vi "GUITest.vi"() -> ()   [LabVIEW 2021]
uses:
  <vilib>/Analysis/1siggen.llb/Ramp Pattern by Samples.vi
  <vilib>/Analysis/NI_AALBase.lvlib
panel:
  out "XY Graph":T1(graph)
  out "element":dbl
  out "Ramp Pattern":dbl[](array[numeric])
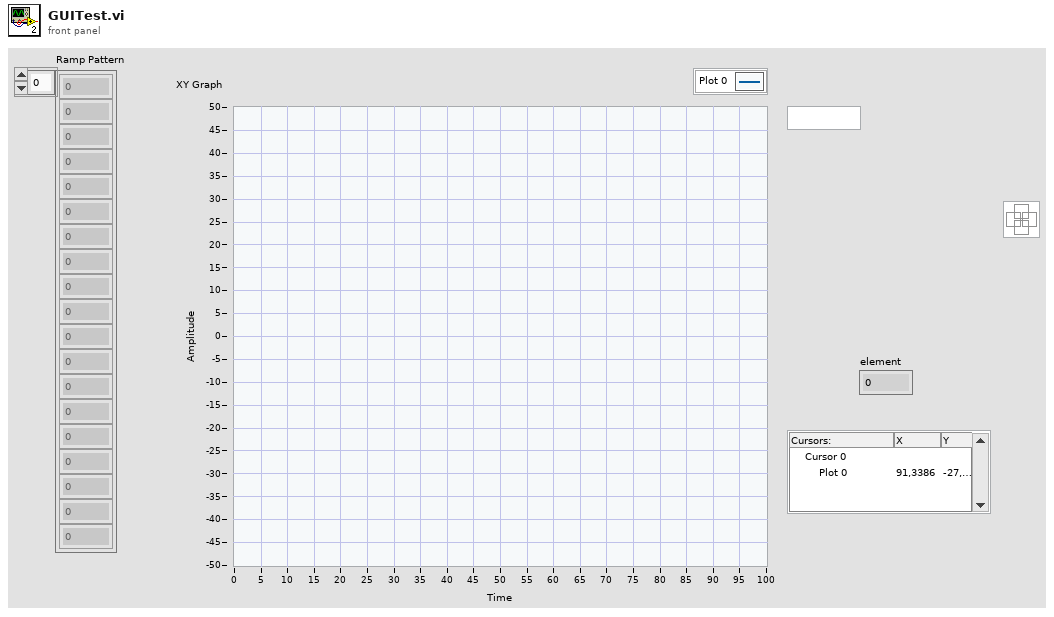
[diagram p1: front panel]
types:
  T1 = cluster{"Ramp Pattern":dbl[], "Sinusoidal Pattern":dbl[]}
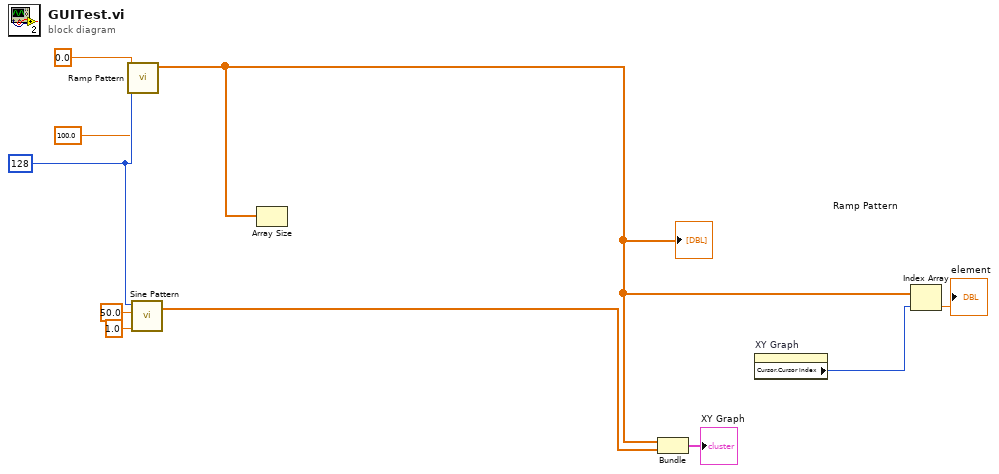
[diagram p0: block diagram]
diagram:
  w9 = 128 ("samples")
  n1 = call-poly <vilib>:"Ramp Pattern.vi"("start"=0.0, "end"=100.0, "samples"=w9) -> ("Ramp Pattern"=w3:dbl[])  [unwired: 7 in, 1 out]
  "Ramp Pattern" <- w3
  n2 = call <vilib>:"Sine Pattern.vi"("cycles"=1.0, "amplitude"=50.0, "samples"=w9) -> ("Sinusoidal Pattern"=w2:dbl[])  [unwired: 1 in, 1 out]
  n3 = Array Size(array=w3) -> ()  [unwired: 1 out]
  n4 = Bundle("Ramp Pattern"=w3, "Sinusoidal Pattern"=w2) -> (→"XY Graph":T1)  [unwired: 1 in]
  n5 = property on="XY Graph" class="XYGraph (strict)"() -> ("Cursor.Cursor Index"=w1:i32)  [unwired: 2 in, 2 out]
  n6 = Index Array(array=w3, index=w1) -> (element=→"element":dbl)
